vi "Stop Impl.vi"(11 "Power Meter in":refnum<class "Power Meter.lvclass">) -> (3 "Power Meter out":refnum<class "Power Meter.lvclass">)   [LabVIEW 2023, in "Power Meter.lvlib" / "Power Meter.lvclass"]
uses:
  Power Meter.lvclass
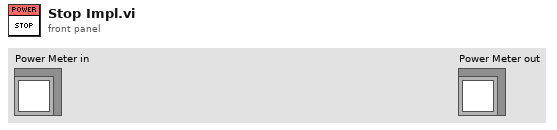
[diagram p1: front panel]
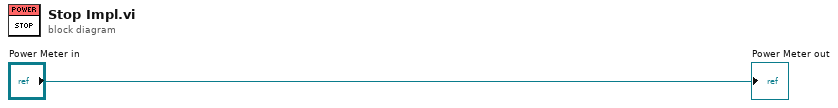
[diagram p0: block diagram]
diagram:
  "Power Meter out" <- "Power Meter in"
